vi "Emit.vi"(8 "error in (no error)":errorcluster, 10 "response":T1, 11 "EventResponder in":refnum<class "EventResponder.lvclass">) -> (0 "error out":errorcluster, 3 "EventResponder out":refnum<class "EventResponder.lvclass">)   [LabVIEW 2013, in "EventResponder.lvclass"]
doc: "Emit a response to the owning application"
uses:
  EventResponder.lvclass
  response.ctl
  driver_status.ctl
  EventResponder.lvclass/EventResponder.ctl
  BaseResponder/BaseResponder.lvclass
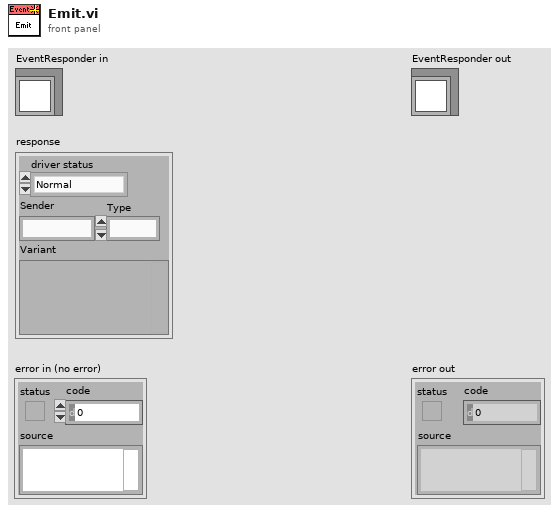
[diagram p1: front panel]
types:
  T1 = typedef "response.ctl" = cluster{"driver status":T2, "Sender":string, "Type":i32, "Variant":variant}
  T2 = typedef "driver_status.ctl" = enum16{"Normal", "Startup", "Connection lost", "Reconnected", "Timeout", "Idle", "Busy"}
  T3 = typedef "response_event.ctl" = refnum<user-event>
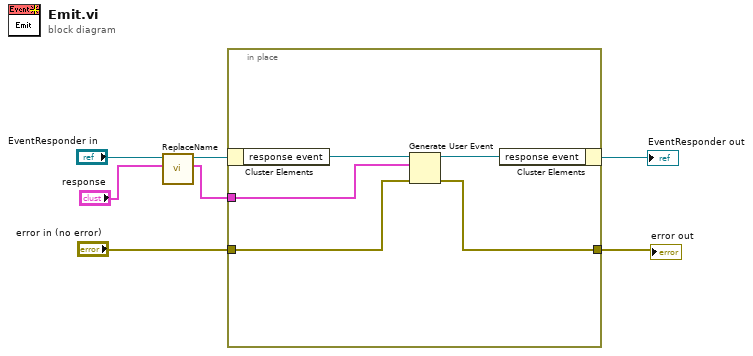
[diagram p0: block diagram]
diagram:
  n1 = call "ReplaceName.vi"("response"="response", "BaseResponder in"="EventResponder in") -> ("response out"=w4:T1, "BaseResponder out"=w5:refnum<class "EventResponder.lvclass">)  [unwired: 7 in, 1 out]
  n2 = in-place "In Place Element Structure" {
    in-place-border: w4 -> [w8]
    in-place-border: "error in (no error)" -> [w9]
    in-place-border: [w10] -> w1
    n3 = in-place-cluster #1(w5) -> ("response event"=w12:T3)
    n4 = Generate User Event(user event=w12, event data cluster=w8, error in=w9) -> (user event out=w11:T3, error out=w10:errorcluster)  [unwired: 1 in]
    n5 = in-place-cluster #1("response event"=w11) -> (→"EventResponder out":refnum<class "EventResponder.lvclass">)
  }
  "error out" <- w1
